vi "somma roi 3d.vi"(9 "ROIs Min Max":dbl[][](array[numeric]), 10 "Data Loaded":dbl[][](array[numeric])) -> (1 "ROIs Array Out":dbl[](array[numeric]))   [LabVIEW 2020]
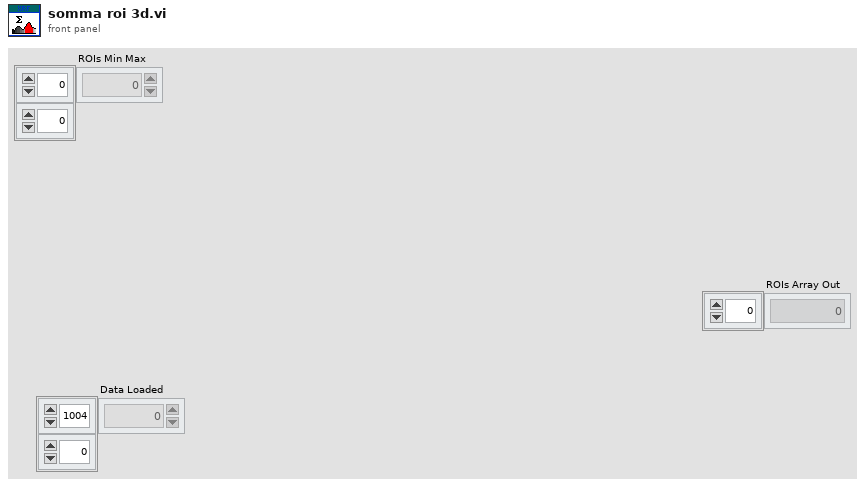
[diagram p1: front panel]
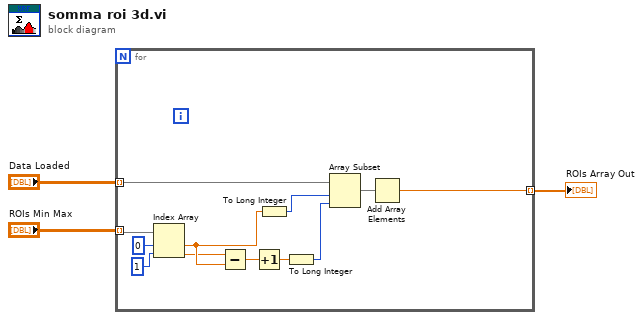
[diagram p0: block diagram]
diagram:
  n1 = for {
    tunnel: "ROIs Min Max" -> [w15] mode=indexing
    tunnel: "Data Loaded" -> [w5] mode=indexing
    tunnel: [w4] -> w1 mode=indexing
    n2 = Index Array(array=w15, index #1=0 ("index"), index #2=1 ("index")) -> (element #1=w10:dbl, element #2=w9:dbl)
    n3 = Subtract(x=w9, y=w10) -> (x-y=w12:dbl)
    n4 = Increment(x=w12) -> (x+1=w11:dbl)
    n5 = To Long Integer(number=w10) -> (32bit integer=w8:i32)
    n6 = To Long Integer(number=w11) -> (32bit integer=w7:i32)
    n7 = Array Subset(array=w5, index=w8, length=w7) -> (w6:dbl[])
    n8 = Add Array Elements(numeric array=w6) -> (sum=w4:dbl)
  }
  "ROIs Array Out" <- w1
